vi "Add Certificate Paths.vi"(10 "Connection Configuration In":T1) -> (2 "Connection Configuration Out":T1)   [LabVIEW 2013, in "OPC UA Client Tests.lvlib"]
doc: "Add Certificate paths to module configuration"
uses:
  OPC UA Client Tests.lvlib
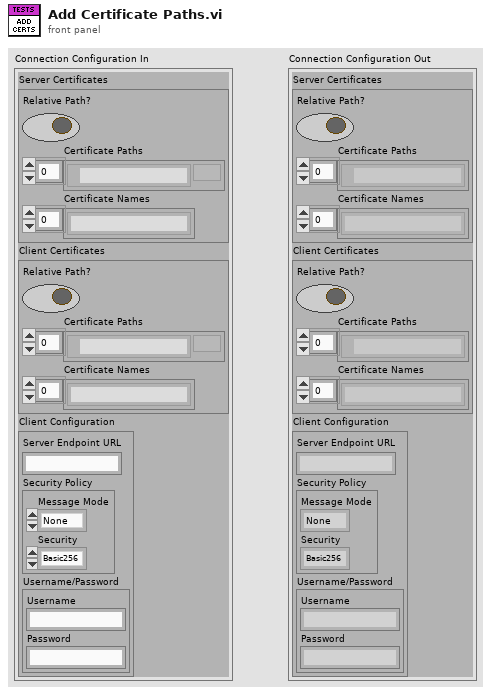
[diagram p1: front panel]
types:
  T1 = cluster{"Server Certificates":cluster{"Relative Path?":bool, "Certificate Paths":path[], "Certificate Names":string[]}, "Client Certificates":cluster{"Relative Path?":bool, "Certificate Paths":path[], "Certificate Names":string[]}, "Client Configuration":cluster{"Server Endpoint URL":string, "Security Policy":cluster{"Message Mode":enum16{"None", "Sign", "Sign and Encrypt"}, "Security":enum16{"Basic256", "Basic128Rsa15"}}, "Username/Password":cluster{"Username":string, "Password":string}}}
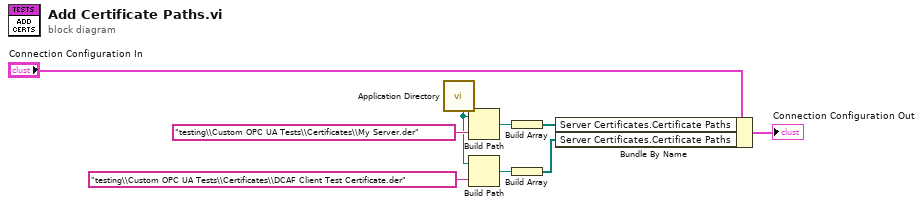
[diagram p0: block diagram]
diagram:
  n1 = call <vilib>:"Application Directory.vi"() -> ("Application Directory"=w3:path)
  n2 = Build Path(base path=w3, name or relative path="testing\\Custom OPC UA Tests\\Certificates\\My Server.der") -> (appended path=w6:path)
  n3 = Build Path(base path=w3, name or relative path="testing\\Custom OPC UA Tests\\Certificates\\DCAF Client Test Certificate.der") -> (appended path=w8:path)
  n4 = Build Array(w6) -> (w7:path[])
  n5 = Build Array(w8) -> (w9:path[])
  n6 = Bundle By Name(cluster="Connection Configuration In", "Server Certificates.Certificate Paths"=w7, "Server Certificates.Certificate Paths"=w9) -> (→"Connection Configuration Out":T1)
